vi "Worked Example--Trapezoidal Rule_ver0.vi"() -> ()   [LabVIEW 2011]
panel:
  out "Approx. Integral":dbl=7.8845418102876925
  out "Waveform Graph":cluster{"Lower limit \"a\"":dbl, dbl, dbl[]}(graph)={"Lower limit \"a\""=0.0, 0.00042, array[10001 elements]}
  in  "Divisions \"N\"":dbl=10000.0
  in  "Upper limit \"b\"":dbl=4.2
  in  "Lower limit \"a\"":dbl
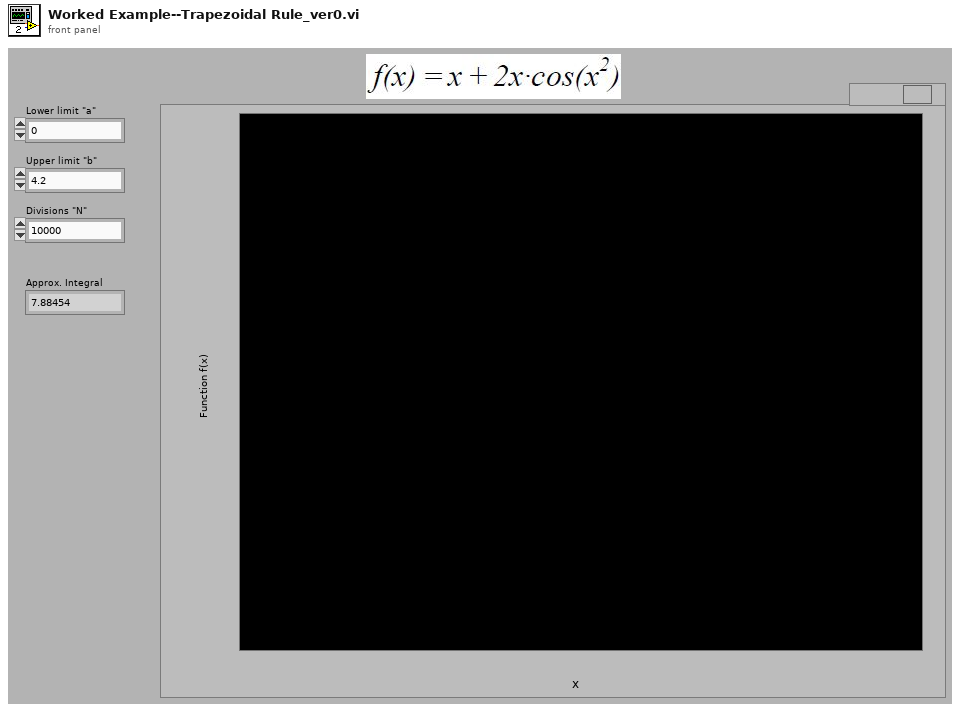
[diagram p1: front panel]
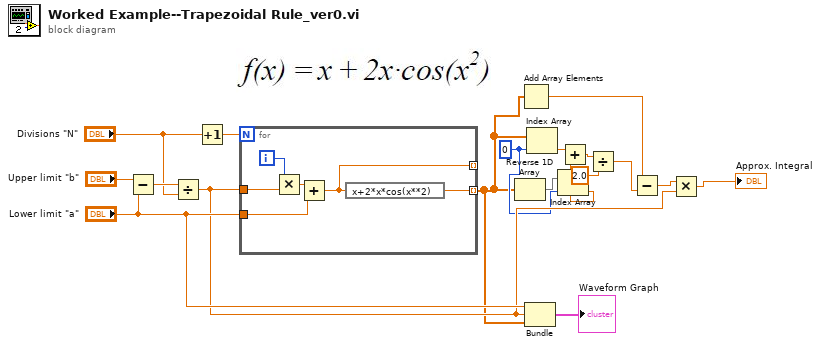
[diagram p0: block diagram]
diagram:
  w3 = 0 ("index")
  n1 = Subtract(x="Upper limit \"b\"", y="Lower limit \"a\"") -> (x-y=w17:dbl)
  n2 = Divide(x=w17, y="Divisions \"N\"") -> (x/y=w8:dbl)
  n3 = Increment(x="Divisions \"N\"") -> (x+1=w13:dbl)
  n4 = for {
    N: w13 -> [_]
    tunnel: w8 -> [w23]
    tunnel: "Lower limit \"a\"" -> [w21]
    tunnel: [w20] -> w1 mode=indexing
    tunnel: [w19] -> _ mode=indexing
    i -> [w24]
    n5 = Multiply(x=w24, y=w23) -> (x*y=w22:dbl)
    n6 = Add(x=w22, y=w21) -> (x+y=w19:dbl)
    n7 = expression code="x+2*x*cos(x**2)"(w19) -> (w20:dbl)
  }
  n8 = Reverse 1D Array(array=w1) -> (reversed array=w4:dbl[])
  n9 = Add Array Elements(numeric array=w1) -> (sum=w5:dbl)
  n10 = Bundle("Lower limit \"a\""="Lower limit \"a\"", w8, w1) -> (→"Waveform Graph":cluster{"Lower limit \"a\"":dbl, dbl, dbl[]})  [unwired: 1 in]
  n11 = Index Array(array=w1, index=w3) -> (element=w12:dbl)
  n12 = Index Array(array=w4, index=w3) -> (element=w2:dbl)
  n13 = Add(x=w12, y=w2) -> (x+y=w10:dbl)
  n14 = Divide(x=w10, y=2.0) -> (x/y=w9:dbl)
  n15 = Subtract(x=w5, y=w9) -> (x-y=w7:dbl)
  n16 = Multiply(x=w7, y=w8) -> (x*y=→"Approx. Integral":dbl)
